vi "calc.vi"(11 "Inputs":T6) -> (3 "Outputs":T1)   [LabVIEW 2013]
uses:
  inputs.ctl
  drive/drive_inputs.ctl
  flinger/flinger_inputs.ctl
  roller/roller_inputs.ctl
  outputs.ctl
  drive/drive_outputs.ctl
  flinger/flinger_outputs.ctl
  <vilib>/Rock Robotics/WPI/Solenoid/WPI_SolenoidValue.ctl
  roller/roller_outputs.ctl
panel:
  in  "Outputs 2":T1
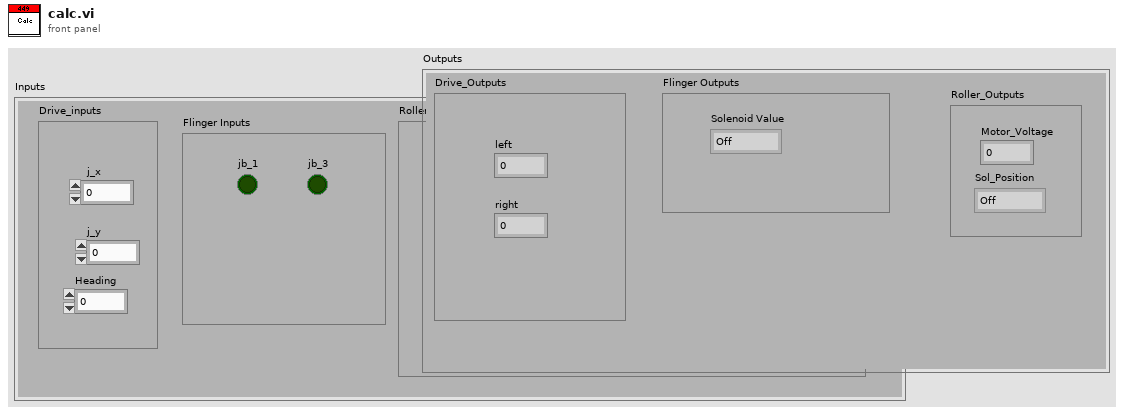
[diagram p1: front panel]
types:
  T1 = typedef "outputs.ctl" = cluster{"Drive_Outputs":T2, "Flinger Outputs":T3, "Roller_Outputs":T5}
  T2 = typedef "drive_outputs.ctl" = cluster{"left":dbl, "right":dbl}
  T3 = typedef "flinger_outputs.ctl" = cluster{"Solenoid Value":T4}
  T4 = typedef "WPI_SolenoidValue.ctl" = enum16{"Off", "On", "Forward", "Reverse"}
  T5 = typedef "roller_outputs.ctl" = cluster{"Sol_Position":T4, "Motor_Voltage":dbl}
  T6 = typedef "inputs.ctl" = cluster{"Drive_inputs":T7, "Flinger Inputs":T8, "Roller Inputs":T9}
  T7 = typedef "drive_inputs.ctl" = cluster{"j_x":dbl, "j_y":dbl, "Heading":dbl}
  T8 = typedef "flinger_inputs.ctl" = cluster{"jb_1":bool, "jb_3":bool}
  T9 = typedef "roller_inputs.ctl" = cluster{"Arm_In":bool, "Motor_On":bool, "Motor_Velocity":dbl}
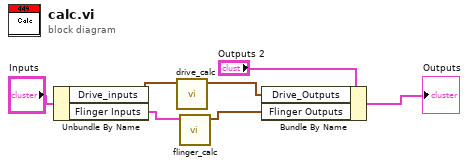
[diagram p0: block diagram]
diagram:
  n1 = Unbundle By Name("Inputs") -> ("Drive_inputs"=w4:T7, "Flinger Inputs"=w2:T8)
  n2 = call "drive_calc.vi"("Drive_inputs"=w4) -> ("Drive_Outputs"=w3:T2)  [unwired: 10 in]
  n3 = call "flinger_calc.vi"("Flinger Inputs"=w2) -> ("Flinger Outputs"=w1:T3)  [unwired: 10 in]
  n4 = Bundle By Name(cluster="Outputs 2", "Drive_Outputs"=w3, "Flinger Outputs"=w1) -> (→"Outputs":T1)
